vi "_Main_02.vi"() -> ()   [LabVIEW 2017]
uses:
  <vilib>/Instr/_visa.llb/VISA Configure Serial Port (Instr).vi
panel:
  out "preforce":dbl
  in  "y":dbl
  out "force":dbl format="%.2f"
  out "Set temp 2":dbl
  in  "Set temp":dbl
  in  "OK Button":bool
  out "TrigTimer, s":dbl
  out "temp":dbl format="%#.2g"
  out "serv1":i32
  out "serv2":i32
  out "serv3":i32
  out "serv4":i32
  out "Vout, V":dbl format="%#.2g"
  out "Vin, V":dbl format="%#.3g"
  out "Temp, K":dbl
  out "Temp_sp, K":dbl
  out "Temp_gsp, K":dbl
  out "Field LOG":cluster{dbl[], dbl[]}(graph)
  out "Bytes at Port":u32
  out "RecTry":i32
  in  "Stop Button":bool
  in  "COM port":refnum<visa-resource-name>
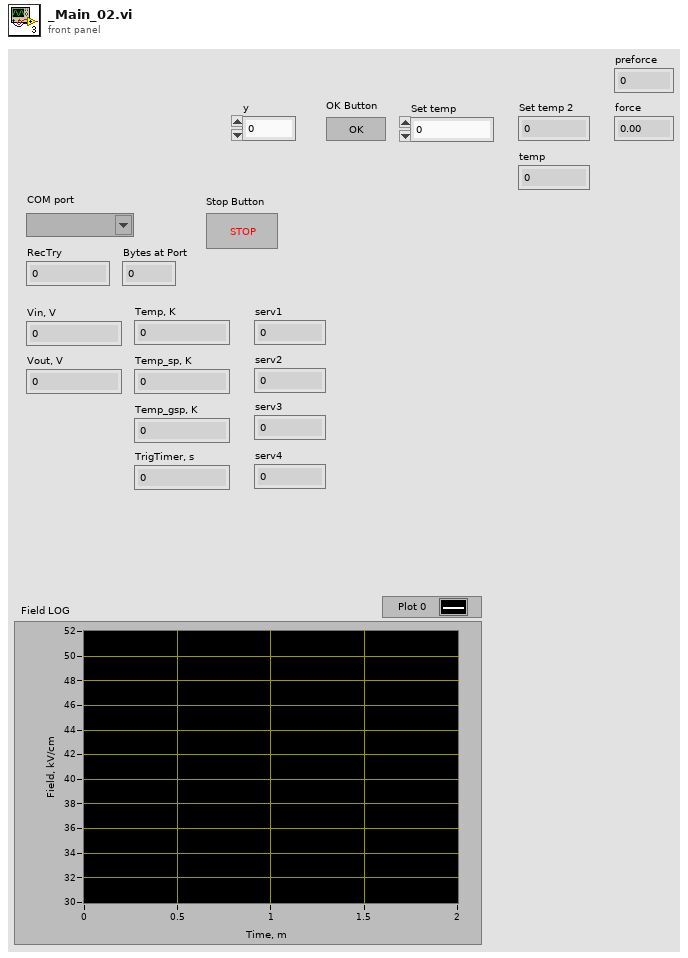
[diagram p1: front panel]
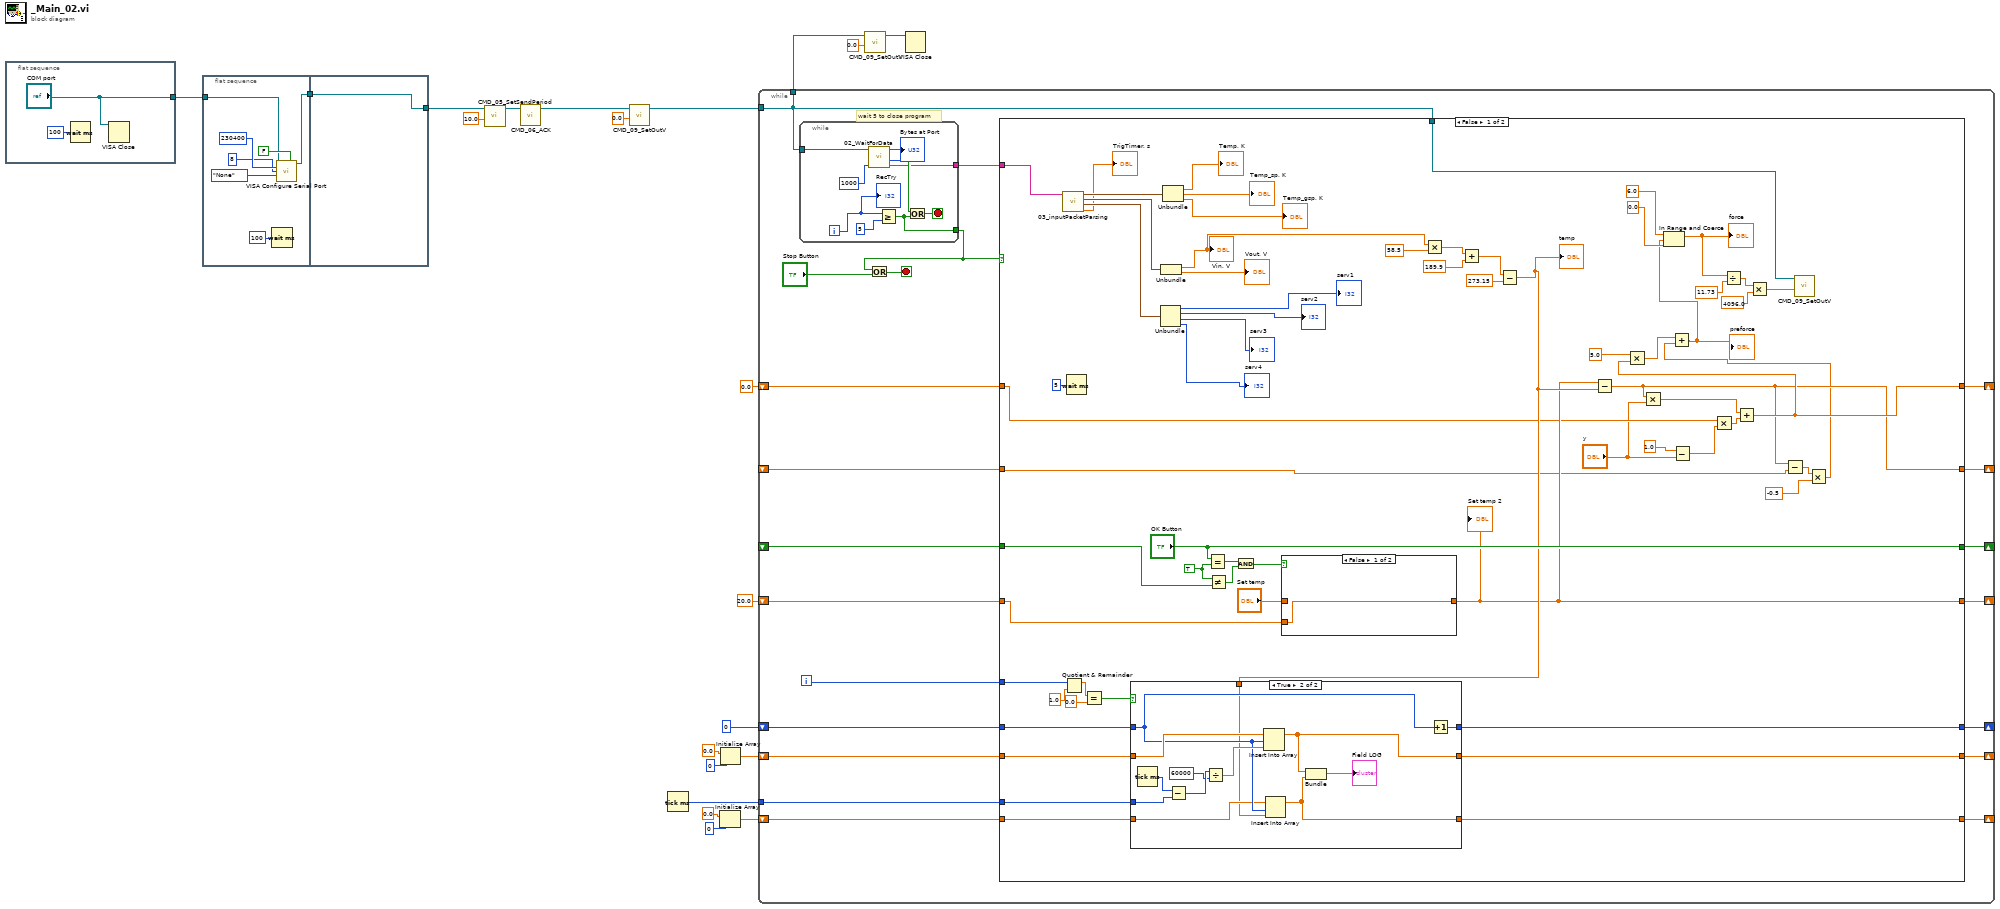
[diagram p0: block diagram]
diagram:
  n1 = flat-sequence {
    tunnel: ["COM port"] -> w21
    frame #0 {
      n2 = Wait (ms)(milliseconds to wait=u32 100) -> ()  [unwired: 1 out]
      n3 = VISA Close(VISA resource name="COM port") -> ()  [unwired: 1 in, 1 out]
    }
  }
  n4 = flat-sequence {
    tunnel: w21 -> [w26]
    tunnel: [w25] -> w18
    tunnel: [w31] -> w9
    tunnel: w18 -> [w31]
    frame #0 {
      n5 = Wait (ms)(milliseconds to wait=u32 100) -> ()  [unwired: 1 out]
      n6 = call-poly "VISA Configure Serial Port"("VISA resource name"=w26, "Enable Termination\nChar (T)"=FALSE ("Enable Termination\nChar (T)"), "baud rate (9600)"=u32 230400, "data bits (8)"=u16 8, "parity (0:none)"=enum16{"None", "Odd", "Even", "Mark", "Space"}."None") -> ("VISA resource name out"=w25:refnum<visa-resource-name>)  [unwired: 9 in, 1 out]
    }
    frame #1 {
    }
  }
  n7 = call "CMD_05_SetSendPeriod.vi"("Period, ms"=10.0, "VISA resource name"=w9) -> ("VISA resource name out"=w19:refnum<visa-resource-name>)  [unwired: 9 in]
  n8 = call "CMD_06_ACK.vi"("VISA resource name"=w19) -> ("VISA resource name out"=w3:refnum<visa-resource-name>)  [unwired: 10 in]
  n9 = call "CMD_09_SetOutV.vi"("Voltage, d"=0.0, "VISA resource name"=w3) -> ("VISA resource name out"=w4:refnum<visa-resource-name>)  [unwired: 9 in]
  n10 = Tick Count (ms)() -> (millisecond timer value=w13:u32)
  n11 = Initialize Array(0.0 ("element"), 0 ("dimension size")) -> (w10:dbl[])
  n12 = Initialize Array(0.0 ("element"), 0 ("dimension size")) -> (w14:dbl[])
  n13 = while {
    tunnel: w4 -> [w38]
    tunnel: [w38] -> w7
    shift-right: [w47] -> _
    shift-left: 0 -> [w48]
    tunnel: w13 -> [w45]
    shift-right: [w43] -> _
    shift-left: w14 -> [w46]
    shift-right: [w42] -> _
    shift-left: w10 -> [w44]
    shift-right: [w40] -> _
    shift-left: _ -> [w39]
    shift-right: [w37] -> _
    shift-left: 20.0 ("Set temp") -> [w36]
    shift-right: [w35] -> _
    shift-left: 0.0 -> [w34]
    shift-right: [w33] -> _
    shift-left: _ -> [w32]
    i -> [w49]
    stop <- w52 stop-if-true
    # "wait 5 to close program"
    n14 = while {
      tunnel: w38 -> [w143]
      tunnel: [w146] -> w51
      tunnel: [w147] -> w50
      i -> [w145]
      stop <- w149 stop-if-true
      n15 = call "02_WaitForData.vi"("WaitTimeoutMS"=u32 1000, "VISA"=w143) -> ("Buffer"=w147:string, "Bytes at Port"=→"Bytes at Port":u32, "Data Recived"=w148:bool)  [unwired: 7 in]
      n16 = Greater Or Equal?(x=w145, y=5) -> (x >= y?=w146:bool)
      n17 = Or(x=w148, y=w146) -> (x .or. y?=w149:bool)
      "RecTry" <- w145
    }
    n18 = Or(x=w51, y="Stop Button") -> (x .or. y?=w52:bool)
    n19 = case shown="False" w51 {
      tunnel: w50 -> [w108 _]
      tunnel: w49 -> [w114 _]
      tunnel: w38 -> [w74 _]
      tunnel: w48 -> [w112 w142]
      tunnel: [w111 w142] -> w47
      tunnel: w46 -> [w89 w141]
      tunnel: w45 -> [w110 _]
      tunnel: w44 -> [w87 w140]
      tunnel: [w109 w141] -> w43
      tunnel: [w60 w140] -> w42
      tunnel: ["OK Button" w139] -> w40
      tunnel: w39 -> [w84 w139]
      tunnel: [w68 w138] -> w37
      tunnel: w36 -> [w76 w138]
      tunnel: [w61 w137] -> w35
      tunnel: w34 -> [w66 w137]
      tunnel: [w59 w136] -> w33
      tunnel: w32 -> [w58 w136]
      frame False {
        w83 = TRUE ("x")
        n20 = call "03_inputPacketParsing.vi"("string"=w108) -> ("TrigTimer, s"=→"TrigTimer, s":dbl, "Service"=w100:cluster{i32, i32, i32, i32}, "Voltage"=w102:cluster{dbl, dbl}, "Temp"=w106:cluster{dbl, dbl, dbl})  [unwired: 7 in]
        n21 = Quotient & Remainder(x=w114, y=1.0) -> (x-y*floor(x/y)=w117:dbl)  [unwired: 1 out]
        n22 = Wait (ms)(milliseconds to wait=u32 5) -> ()  [unwired: 1 out]
        n23 = Equal?(x=w117, y=0.0) -> (x = y?=w113:bool)
        n24 = Unbundle(w100) -> (→"serv1":i32, →"serv2":i32, →"serv3":i32, →"serv4":i32)
        n25 = Unbundle(w102) -> (w95:dbl, →"Vout, V":dbl)
        "Vin, V" <- w95
        n26 = Unbundle(w106) -> (→"Temp, K":dbl, →"Temp_sp, K":dbl, →"Temp_gsp, K":dbl)
        n27 = Equal?(x="OK Button", y=w83) -> (x = y?=w86:bool)
        n28 = Not Equal?(x=w83, y=w84) -> (x != y?=w82:bool)
        n29 = And(x=w86, y=w82) -> (x .and. y?=w81:bool)
        n30 = case shown="False" w81 {
          tunnel: "Set temp" -> [_ w119]
          tunnel: [w118 w119] -> w68
          tunnel: w76 -> [w118 _]
          frame False {
          }
          frame True {
          }
        }
        "Set temp 2" <- w68
        n31 = Multiply(x=w95, y=58.5) -> (x*y=w93:dbl)
        n32 = Add(x=w93, y=189.9) -> (x+y=w91:dbl)
        n33 = Subtract(x=w91, y=273.15) -> (x-y=w73:dbl)
        "temp" <- w73
        n34 = case shown="True" w113 {
          tunnel: w112 -> [w122 w128]
          tunnel: [w122 w131] -> w111
          tunnel: w89 -> [w120 w129]
          tunnel: w110 -> [_ w134]
          tunnel: w87 -> [w121 w127]
          tunnel: [w121 w125] -> w60
          tunnel: [w120 w124] -> w109
          tunnel: w73 -> [_ w123]
          frame False {
          }
          frame True {
            n35 = Tick Count (ms)() -> (millisecond timer value=w135:u32)
            n36 = Subtract(x=w135, y=w134) -> (x-y=w133:u32)
            n37 = Divide(x=w133, y=u32 60000) -> (x/y=w130:dbl)
            n38 = Insert Into Array(array=w129, index=w128, new element=w130) -> (w124:dbl[])
            n39 = Insert Into Array(array=w127, index=w128, new element=w123) -> (w125:dbl[])
            n40 = Bundle(w124, w125) -> (→"Field LOG":cluster{dbl[], dbl[]})  [unwired: 1 in]
            n41 = Increment(x=w128) -> (x+1=w131:i32)
          }
        }
        n42 = Subtract(x=w68, y=w73) -> (x-y=w59:dbl)
        n43 = Multiply(x=w59, y="y") -> (x*y=w63:dbl)
        n44 = Subtract(x=1.0, y="y") -> (x-y=w65:dbl)
        n45 = Multiply(x=w66, y=w65) -> (x*y=w64:dbl)
        n46 = Add(x=w63, y=w64) -> (x+y=w61:dbl)
        n47 = Multiply(x=5.0, y=w61) -> (x*y=w54:dbl)
        n48 = Subtract(x=w59, y=w58) -> (x-y=w57:dbl)
        n49 = Multiply(x=w57, y=-0.5) -> (x*y=w53:dbl)
        n50 = Add(x=w54, y=w53) -> (x+y=w55:dbl)
        "preforce" <- w55
        n51 = In Range and Coerce(upper limit=6.0, x=w55, lower limit=0.0) -> (coerced(x)=w70:dbl)  [unwired: 1 out]
        "force" <- w70
        n52 = Divide(x=w70, y=11.73) -> (x/y=w79:dbl)
        n53 = Multiply(x=w79, y=4096.0) -> (x*y=w75:dbl)
        n54 = call "CMD_09_SetOutV.vi"("Voltage, d"=w75, "VISA resource name"=w74) -> ()  [unwired: 9 in, 1 out]
      }
      frame True {
      }
    }
  }
  n55 = call "CMD_09_SetOutV.vi"("Voltage, d"=0.0, "VISA resource name"=w7) -> ("VISA resource name out"=w8:refnum<visa-resource-name>)  [unwired: 9 in]
  n56 = VISA Close(VISA resource name=w8) -> ()  [unwired: 1 in, 1 out]
